vi "Cursor Object Event.vi"(4 "Cursor Action":enum16{"Update", "Remove", "Nothing"}(ring), 8 "error in (no error)":errorcluster, 9 "Object Cluster In":T3, 10 "Actual Transform In":T1, 11 "3D Plot.lvclass in":refnum<class "3D Plot.lvclass">) -> (0 "error out":errorcluster, 1 "Object Cluster Out":T3, 2 "Actual Transform Out":T1, 3 "3D Plot.lvclass out":refnum<class "3D Plot.lvclass">)   [LabVIEW 2020, in "3D Plot.lvclass"]
uses:
  <vilib>/Math Plots/3D Math Plots/3D Plot/3D Plot/3D Plot.lvclass
  <vilib>/Math Plots/3D Math Plots/3D Plot/3D Plot/Typedef/Object Cluster.ctl
  <vilib>/Math Plots/3D Math Plots/3D Plot/3D Plot/Typedef/Actual Transform.ctl
  <vilib>/Math Plots/3D Math Plots/3D Plot/3D Plot/Typedef/Range Clusters.ctl
  <vilib>/Math Plots/3D Math Plots/3D Plot/3D Plot/3D Plot.lvclass/3D Plot.ctl
  <vilib>/picture/3D Picture Control/Object/Create Object (name).vi
  <vilib>/picture/3D Picture Control/NI_3D Picture Control.lvlib
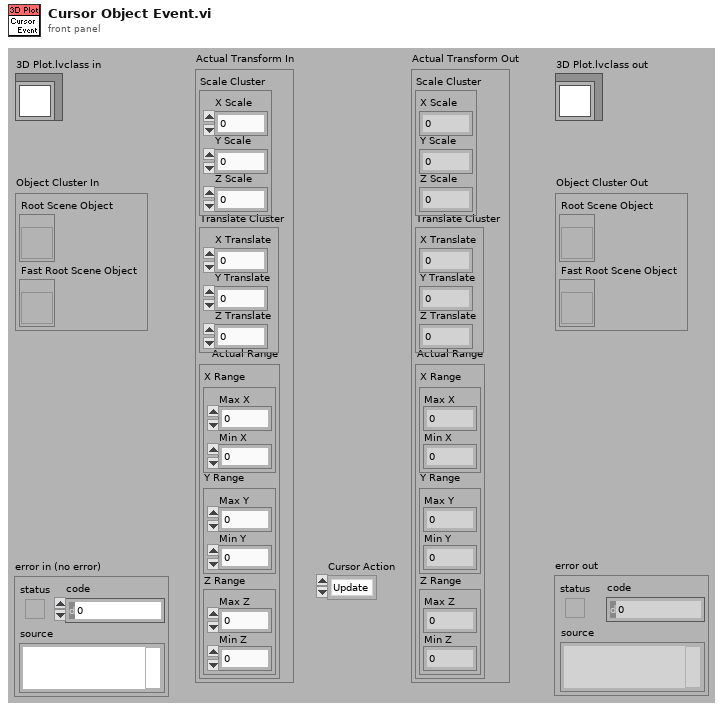
[diagram p1: front panel]
types:
  T1 = typedef "3D Plot.lvclass/Actual Transform.ctl" = cluster{"Scale Cluster":cluster{"X Scale":sgl, "Y Scale":sgl, "Z Scale":sgl}, "Translate Cluster":cluster{"X Translate":sgl, "Y Translate":sgl, "Z Translate":sgl}, "Actual Range":T2}
  T2 = typedef "3D Plot.lvclass/Range Clusters.ctl" = cluster{"X Range":cluster{"Max X":sgl, "Min X":sgl}, "Y Range":cluster{"Max Y":sgl, "Min Y":sgl}, "Z Range":cluster{"Max Z":sgl, "Min Z":sgl}}
  T3 = typedef "3D Plot.lvclass/Object Cluster.ctl" = cluster{"Root Scene Object":refnum<vi>, "Fast Root Scene Object":refnum<vi>}
  T4 = typedef "3D Plot.lvclass/Cursor Property Array.ctl" = T5[]
  T5 = typedef "3D Plot.lvclass/Cursor Property.ctl" = cluster{"Cursor Visible":bool, "Cursor Enable":bool, "Cursor Position":T6, "Cursor Point":T7, "Cursor Line":T9, "Cursor Plane":T11, "Cursor Text":T12}
  T6 = typedef "3D Plot.lvclass/Cursor Position.ctl" = cluster{"Cursor Plot ID":i32, "Cursor X":sgl, "Cursor Y":sgl, "Cursor Z":sgl, "Cursor Snap To":enum16{"Fixed", "Nearest Plot", "Snap to Plot"}}
  T7 = typedef "3D Plot.lvclass/Cursor Point.ctl" = cluster{"Cursor Point Color":u32, "Cursor Point Size":sgl, "Cursor Point Style":T8}
  T8 = typedef "3D Plot.lvclass/Sprite Type.ctl" = enum16{"None", "Empty Square", "Solid Square", "Empty Diamond", "Solid Diamond", "Empty Circle", "Solid Circle", "Asterisk", "Bold X", "Wireframe Sphere", "Solid Sphere", "Wireframe Cube", "Solid Cube"}
  T9 = typedef "3D Plot.lvclass/Cursor Line.ctl" = cluster{"Cursor Line Color":u32, "Cursor Line Width":sgl, "Cursor Line Style":T10}
  T10 = typedef "3D Plot.lvclass/Line Type.ctl" = enum16{"None", "Solid", "Dash", "Dot", "Dash Dot"}
  T11 = typedef "3D Plot.lvclass/Cursor Plane.ctl" = cluster{"Cursor Plane Color":u32, "Cursor Plane Opacity":sgl, "Draw Cursor Plane X-Z":bool, "Draw Cursor Plane Y-Z":bool, "Draw Cursor Plane X-Y":bool}
  T12 = typedef "3D Plot.lvclass/Cursor Text.ctl" = cluster{"Cursor Text":string, "Cursor Text Size":u16, "Cursor Show Position":bool, "Cursor Show Name":bool, "Cursor Text Color":u32, "Background Color":u32, "Background Opacity":sgl}
  T13 = typedef "3D Plot.lvclass/Range Property.ctl" = cluster{"Range Cluster":T2, "Auto Range":cluster{"Auto Range X":bool, "Auto Range Y":bool, "Auto Range Z":bool}, "Inverted":cluster{"Inverted X":bool, "Inverted Y":bool, "Inverted Z":bool}, "Logarithm":cluster{"Logarithm X":bool, "Logarithm Y":bool, "Logarithm Z":bool}}
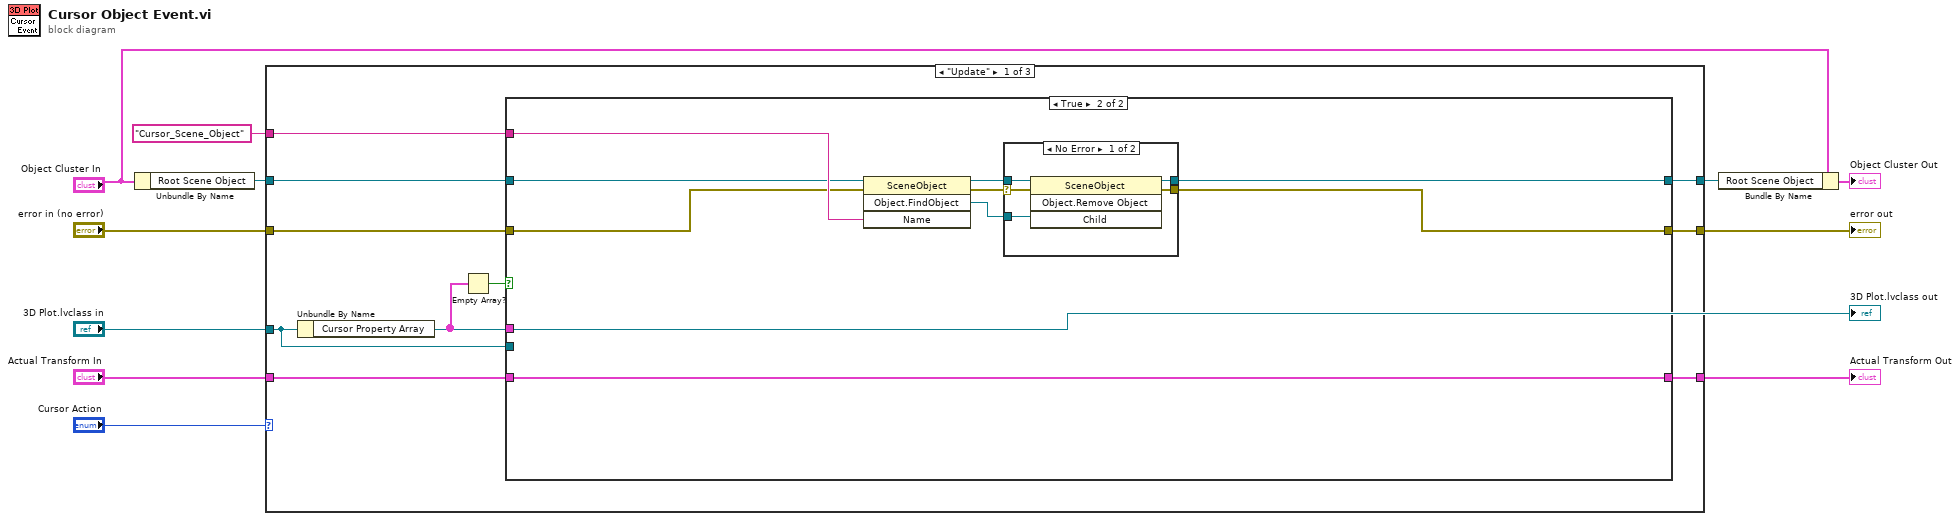
[diagram p0: block diagram]
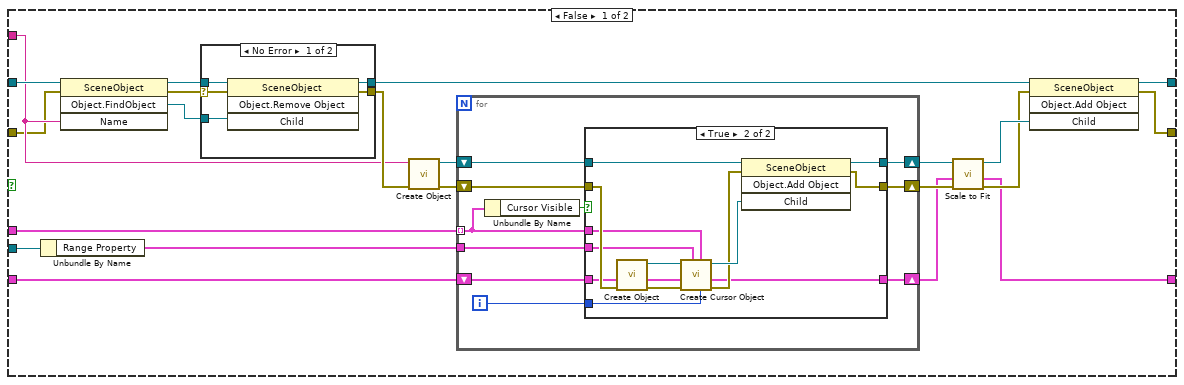
[diagram p2: hidden frame]
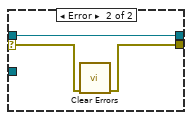
[diagram p3: hidden frame]
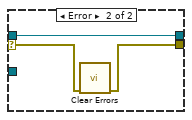
[diagram p5: hidden frame]
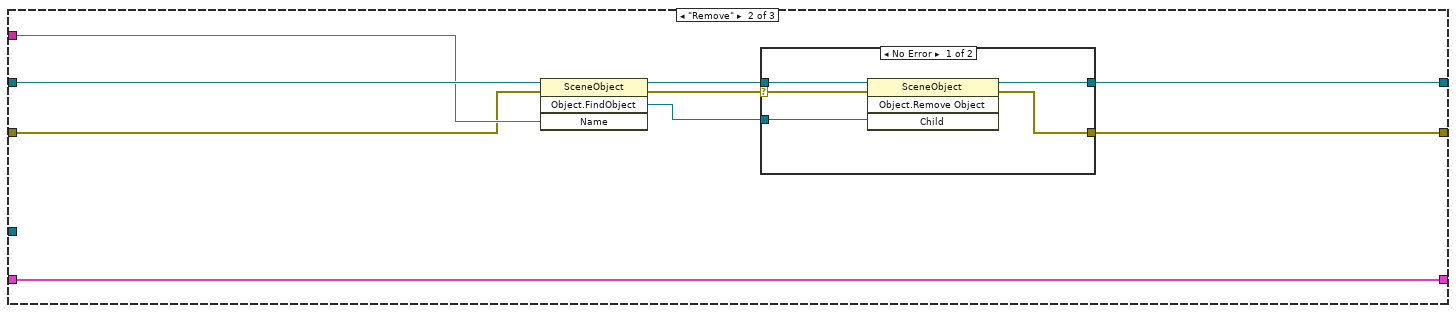
[diagram p6: hidden frame]
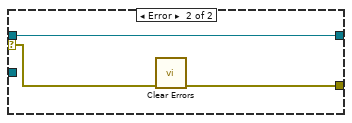
[diagram p7: hidden frame]
diagram:
  n1 = Unbundle By Name("Object Cluster In") -> ("Root Scene Object"=w10:refnum<vi>)
  n2 = case shown="\"Update\"" "Cursor Action" {
    tunnel: w10 -> [w17 w100 w114]
    tunnel: [w21 w103 w114] -> w8
    tunnel: [w20 w102 w113] -> w7
    tunnel: "error in (no error)" -> [w16 w95 w113]
    tunnel: "3D Plot.lvclass in" -> [w13 _ _]
    tunnel: "Actual Transform In" -> [w19 w101 w112]
    tunnel: [w18 w101 w112] -> w3
    tunnel: "Cursor_Scene_Object" ("Name") -> [w15 w97 _]
    frame "Update" {
      n3 = Unbundle By Name(w13) -> ("Cursor Property Array"=w14:T4)
      n4 = Empty Array?(array=w14) -> (empty?=w12:bool)
      n5 = case shown="True" w12 {
        tunnel: [w43 w80] -> w21
        tunnel: [w40 w78] -> w20
        tunnel: w19 -> [w34 w86]
        tunnel: [w33 w86] -> w18
        tunnel: w17 -> [w32 w81]
        tunnel: w16 -> [w23 w79]
        tunnel: w15 -> [w27 w82]
        tunnel: w14 -> [w26 _]
        tunnel: w13 -> [w25 _]
        frame False {
          n6 = Unbundle By Name(w25) -> ("Range Property"=w24:T13)
          n7 = invoke class="SceneObject" method="Object.FindObject"(reference=w32, error in=w23, "Name"=w27) -> (reference out=w29:refnum<vi>, error out=w22:errorcluster, "FindObject"=w28:refnum<vi>)  [unwired: 1 in, 1 out]
          n8 = case shown="No Error" w22 {
            selector: w22 -> [w44 w50]
            tunnel: [w46 w49] -> w30
            tunnel: w29 -> [w48 w51]
            tunnel: w28 -> [w47 _]
            tunnel: [w45 w51] -> w31
            frame No Error {
              n9 = invoke class="SceneObject" method="Object.Remove Object"(reference=w48, error in=w44, "Child"=w47) -> (reference out=w45:refnum<vi>, error out=w46:errorcluster)  [unwired: 1 in, 2 out]
            }
            frame Error {
              n10 = call <vilib>:"Clear Errors.vi"("error in (no error)"=w50) -> ("error out"=w49:errorcluster)  [unwired: 5 in, 1 out]
            }
          }
          n11 = call-poly <vilib>:"Create Object.vi"("error in (no error)"=w30, "Name"=w27) -> ("error out"=w41:errorcluster, "Scene:New Object"=w42:refnum<vi>)  [unwired: 8 in]
          n12 = for {
            tunnel: w26 -> [w58] mode=indexing
            shift-right: [w60] -> w39
            shift-left: w42 -> [w61]
            shift-right: [w56] -> w36
            shift-left: w41 -> [w57]
            shift-right: [w54] -> w35
            shift-left: w34 -> [w53]
            tunnel: w24 -> [w55]
            i -> [w52]
            n13 = Unbundle By Name(w58) -> ("Cursor Visible"=w59:bool)
            n14 = case shown="True" w59 {
              tunnel: w61 -> [w64 w76]
              tunnel: [w64 w77] -> w60
              tunnel: w58 -> [_ w67]
              tunnel: w57 -> [w63 w75]
              tunnel: [w63 w74] -> w56
              tunnel: w55 -> [_ w66]
              tunnel: w53 -> [w62 w69]
              tunnel: [w62 w68] -> w54
              tunnel: w52 -> [_ w65]
              frame False {
              }
              frame True {
                n15 = call-poly <vilib>:"Create Object.vi"("error in (no error)"=w75) -> ("error out"=w70:errorcluster, "Scene:New Object"=w73:refnum<vi>)  [unwired: 9 in]
                n16 = call <vilib>:"Create Cursor Object.vi"("Cursor ID"=w65, "Cursor Property"=w67, "Range Property"=w66, "error in (no error)"=w70, "Actual Transform In"=w69, "Cursor Object In"=w73) -> ("error out"=w71:errorcluster, "Actual Transform Out"=w68:T1, "Cursor Object Out"=w72:refnum<vi>)  [unwired: 1 in, 2 out]
                n17 = invoke class="SceneObject" method="Object.Add Object"(reference=w76, error in=w71, "Child"=w72) -> (reference out=w77:refnum<vi>, error out=w74:errorcluster)  [unwired: 1 in, 2 out]
              }
            }
          }
          n18 = call <vilib>:"Scale to Fit.vi"("error in (no error)"=w36, "Actual Transform In"=w35, "Plot Object In"=w39) -> ("error out"=w37:errorcluster, "Actual Transform Out"=w33:T1, "Plot Object Out"=w38:refnum<vi>)  [unwired: 6 out]
          n19 = invoke class="SceneObject" method="Object.Add Object"(reference=w31, error in=w37, "Child"=w38) -> (reference out=w43:refnum<vi>, error out=w40:errorcluster)  [unwired: 1 in, 2 out]
        }
        frame True {
          n20 = invoke class="SceneObject" method="Object.FindObject"(reference=w81, error in=w79, "Name"=w82) -> (reference out=w85:refnum<vi>, error out=w83:errorcluster, "FindObject"=w84:refnum<vi>)  [unwired: 1 in, 1 out]
          n21 = case shown="No Error" w83 {
            selector: w83 -> [w87 w93]
            tunnel: [w89 w92] -> w78
            tunnel: w85 -> [w91 w94]
            tunnel: w84 -> [w90 _]
            tunnel: [w88 w94] -> w80
            frame No Error {
              n22 = invoke class="SceneObject" method="Object.Remove Object"(reference=w91, error in=w87, "Child"=w90) -> (reference out=w88:refnum<vi>, error out=w89:errorcluster)  [unwired: 1 in, 2 out]
            }
            frame Error {
              n23 = call <vilib>:"Clear Errors.vi"("error in (no error)"=w93) -> ("error out"=w92:errorcluster)  [unwired: 5 in, 1 out]
            }
          }
        }
      }
    }
    frame "Remove" {
      n24 = invoke class="SceneObject" method="Object.FindObject"(reference=w100, error in=w95, "Name"=w97) -> (reference out=w99:refnum<vi>, error out=w96:errorcluster, "FindObject"=w98:refnum<vi>)  [unwired: 1 in, 1 out]
      n25 = case shown="No Error" w96 {
        selector: w96 -> [w104 w110]
        tunnel: w98 -> [w108 _]
        tunnel: w99 -> [w107 w111]
        tunnel: [w106 w111] -> w103
        tunnel: [w105 w109] -> w102
        frame No Error {
          n26 = invoke class="SceneObject" method="Object.Remove Object"(reference=w107, error in=w104, "Child"=w108) -> (reference out=w106:refnum<vi>, error out=w105:errorcluster)  [unwired: 1 in, 2 out]
        }
        frame Error {
          n27 = call <vilib>:"Clear Errors.vi"("error in (no error)"=w110) -> ("error out"=w109:errorcluster)  [unwired: 5 in, 1 out]
        }
      }
    }
    frame "Nothing", Default {
    }
  }
  "error out" <- w7
  "Actual Transform Out" <- w3
  n28 = Bundle By Name(cluster="Object Cluster In", "Root Scene Object"=w8) -> (→"Object Cluster Out":T3)
  "3D Plot.lvclass out" <- "3D Plot.lvclass in"
